vi "Autonomous Independent.vi"   [LabVIEW 2013]
doc: "This VI is called when autonomous begins, and will automatically be terminated when autonomous ends. You can carry out timed or sensor driven robot movement independently without needing to return to the caller."
uses:
  <vilib>/Rock Robotics/WPI/Solenoid/WPI_SolenoidValue.ctl
  Robot Global Data.vi
  <vilib>/Rock Robotics/WPI/RobotDrive/WPI_RobotDriveGetSetRefNum.vi
  <vilib>/Rock Robotics/WPI/Solenoid/WPI_SolenoidSetEnum.vi
  <vilib>/Rock Robotics/WPI/RobotDrive/WPI_RobotDriveArcadeDrive_Standard(NoSaturation).vi
  <vilib>/Rock Robotics/WPI/Solenoid/Deprecated/WPI_SolenoidGetBool.vi
  <vilib>/Rock Robotics/WPI/Joystick/WPI_JoystickGetSetRefNum.vi
panel:
  # "Be sure to right-click and choose Data Operations>>Make Current Value default if you want to save the array values with the VI"
types:
  T1 = typedef "WPI_JoystickDevRef.ctl" = cluster{"Device":T2}
  T2 = typedef "WPI_JoystickDeviceEnum.ctl" = enum16{"USB 1", "USB 2", "USB 3", "USB 4", "Kinect 1", "Kinect 2"}
  T3 = cluster{"axis 1 (x)":dbl, "axis 2 (y)":dbl, "axis 3 (throttle)":dbl, "axis 4":dbl, "axis 5":dbl, "axis 6":dbl}
  T4 = typedef "WPI_MotorControlDeviceRef.ctl" = cluster{"DeviceStatus":errorcluster, "Type":enum16{"PWM", "CAN"}, "PWM":cluster{"Digital Module":T5, "PWM Channel":T6, "DeadBand":T7}, "CAN":cluster{"Device Number":u8, "Control Mode":T8, "Semaphore":T9, "Max Vout":dbl}, "Invert":bool, "TransformRef":T10, "InvTransformRef":T10}
  T5 = typedef "FPGA_TypedefDigitalModule.ctl" = enum16{"Digital Module 1", "Digital Module 2"}
  T6 = typedef "FPGA_DIOPWMChannel.ctl" = enum8{"PWM 1", "PWM 2", "PWM 3", "PWM 4", "PWM 5", "PWM 6", "PWM 7", "PWM 8", "PWM 9", "PWM 10", "Invalid"}
  T7 = typedef "WPI_PWMDeadband.ctl" = cluster{"Name":string, "maxPositivePwm":i32, "minPositivePwm":i32, "centerPwm":i32, "maxNegativePwm":i32, "minNegativePwm":i32, "angularRange":u16}
  T8 = typedef "WPI_CANJaguar_ControlMode.ctl" = enum8{"Percent VBus", "Current", "Speed", "Position", "Voltage"}
  T9 = typedef "Semaphore RefNum" = refnum<k1>
  T10 = typedef "WPI_PWMTransform_ConPane.ctl" = refnum<vi>
  T11 = typedef "WPI_SolenoidDevRef.ctl" = cluster{"DevStatus":errorcluster, "Solenoid Module":T12, "Forward Solenoid Channel":T13, "Reverse Solenoid Channel":T13}
  T12 = typedef "FPGA_TypedefSolenoidModule.ctl" = enum16{"Solenoid Module 1", "Solenoid Module 2"}
  T13 = typedef "WPI_SolenoidChannel.ctl" = enum8{"Solenoid 1", "Solenoid 2", "Solenoid 3", "Solenoid 4", "Solenoid 5", "Solenoid 6", "Solenoid 7", "Solenoid 8", "Invalid"}
  T14 = typedef "WPI_RobotDriveDevRef.ctl" = cluster{"DevStatus":errorcluster, "Motors[]":T4[], "Square Inputs":bool, "Max Output":dbl, "Isochronous":bool}
  T15 = typedef "WPI_SolenoidValue.ctl" = enum16{"Off", "On", "Forward", "Reverse"}
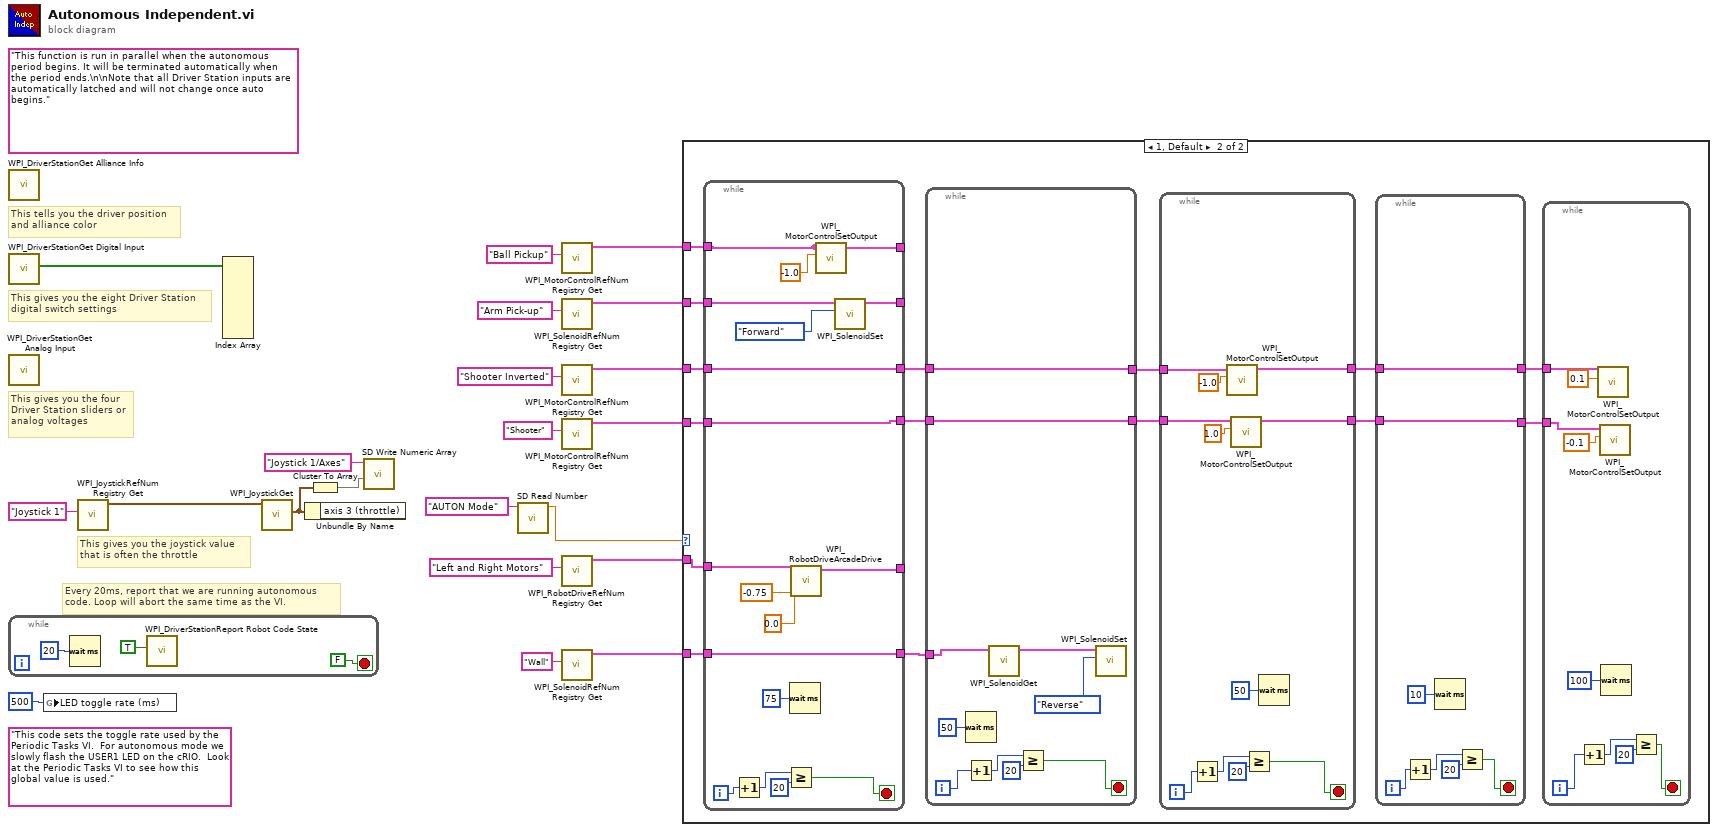
[diagram p0: block diagram]
diagram:
  (unwired) "This code sets the toggle rate used by the Periodic Tasks VI.  For autonomous mode we slowly flash the USER1 LED on the cRIO.  Look at the Periodic Tasks VI to see how this global value is used."
  (unwired) "This function is run in parallel when the autonomous period begins. It will be terminated automatically when the period ends.\n\nNote that all Driver Station inputs are automatically latched and will not change once auto begins."
  # "Every 20ms, report that we are running autonomous\ncode. Loop will abort the same time as the VI."
  # "This gives you the joystick value\nthat is often the throttle"
  # "This tells you the driver position\nand alliance color"
  # "This gives you the eight Driver Station\ndigital switch settings"
  # "This gives you the four\nDriver Station sliders or\nanalog voltages"
  n1 = call <vilib>:"WPI_DriverStationGet Alliance Info.vi"() -> ()  [unwired: 12 out]
  n2 = call <vilib>:"WPI_DriverStationGet Digital Input.vi"() -> ("Driver Station Digital Input (1-8)"=w21:bool[])  [unwired: 11 out]
  n3 = call <vilib>:"WPI_DriverStationGet Analog Input.vi"() -> ()  [unwired: 12 out]
  n4 = while {
    stop <- FALSE stop-if-true
    n5 = Wait (ms)(milliseconds to wait=u32 20) -> ()  [unwired: 1 out]
    n6 = call <vilib>:"WPI_DriverStationReport Robot Code State.vi"("Autonomous"=TRUE) -> ()  [unwired: 10 in, 1 out]
  }
  n7 = global write "Robot Global Data.vi" "LED toggle rate (ms)"(u32 500 ("LED ms toggle rate")) -> ()
  n8 = call <vilib>:"WPI_JoystickRefNum Registry Get.vi"("refnum name"="Joystick 1") -> ("JoystickDevRef"=w19:T1)  [unwired: 1 in, 9 out]
  n9 = Index Array(array=w21) -> ()  [unwired: 8 in, 8 out]
  n10 = call <vilib>:"WPI_JoystickGet.vi"("JoystickDevRef"=w19) -> ("Axes"=w16:T3)  [unwired: 1 in, 5 out]
  n11 = Unbundle By Name(w16) -> ()  [unwired: 1 out]
  n12 = Cluster To Array(cluster=w16) -> (array=w17:dbl[])
  n13 = call <vilib>:"SD Write Numeric Array.vi"("Numeric Array"=w17, "Name"="Joystick 1/Axes") -> ()  [unwired: 8 in, 2 out]
  n14 = call <vilib>:"SD Read Number.vi"("Name"="AUTON Mode") -> ("Numeric"=w13:dbl)  [unwired: 8 in, 2 out]
  n15 = call <vilib>:"WPI_MotorControlRefNum Registry Get.vi"("refnum name"="Ball Pickup") -> ("MotorControlDevRef"=w1:T4)  [unwired: 9 in, 1 out]
  n16 = call <vilib>:"WPI_SolenoidRefNum Registry Get.vi"("refnum name"="Arm Pick-up") -> ("SolenoidDevRef"=w2:T11)  [unwired: 9 in, 1 out]
  n17 = call <vilib>:"WPI_MotorControlRefNum Registry Get.vi"("refnum name"="Shooter Inverted") -> ("MotorControlDevRef"=w3:T4)  [unwired: 9 in, 1 out]
  n18 = call <vilib>:"WPI_MotorControlRefNum Registry Get.vi"("refnum name"="Shooter") -> ("MotorControlDevRef"=w4:T4)  [unwired: 9 in, 1 out]
  n19 = call <vilib>:"WPI_RobotDriveRefNum Registry Get.vi"("refnum name"="Left and Right Motors") -> ("RobotDriveDevRef"=w6:T14)  [unwired: 9 in, 1 out]
  n20 = call <vilib>:"WPI_SolenoidRefNum Registry Get.vi"("refnum name"="Wall") -> ("SolenoidDevRef"=w5:T11)  [unwired: 9 in, 1 out]
  n21 = case shown="1, Default" w13 {
    tunnel: w6 -> [_ w39]
    tunnel: w5 -> [_ w25]
    tunnel: w4 -> [_ w38]
    tunnel: w3 -> [_ w37]
    tunnel: w2 -> [_ w36]
    tunnel: w1 -> [_ w35]
    frame 0 {
    }
    frame 1, Default {
      n22 = while {
        tunnel: w39 -> [w88]
        tunnel: [w86] -> _
        tunnel: [w85] -> w34
        tunnel: w38 -> [w85]
        tunnel: w37 -> [w84]
        tunnel: [w84] -> w33
        tunnel: w36 -> [w79]
        tunnel: w35 -> [w78]
        tunnel: [w78] -> _
        tunnel: [w79] -> _
        tunnel: [w81] -> w26
        tunnel: w25 -> [w81]
        i -> [w92]
        stop <- w89 stop-if-true
        n23 = Increment(x=w92) -> (x+1=w91:i32)
        n24 = Greater Or Equal?(x=w91, y=20) -> (x >= y?=w89:bool)
        n25 = Wait (ms)(milliseconds to wait=u32 75) -> ()  [unwired: 1 out]
        n26 = call-poly <vilib>:"WPI_RobotDriveArcadeDrive.vi"("Y axis value"=-0.75, "X axis value"=0.0, "RobotDriveDevRef"=w88) -> ("RobotDriveDevRef"=w86:T14)  [unwired: 6 in, 2 out]
        n27 = call <vilib>:"WPI_MotorControlSetOutput.vi"("Output"=-1.0, "MotorControlDevRef"=w78) -> ()  [unwired: 7 in, 3 out]
        n28 = call-poly <vilib>:"WPI_SolenoidSet.vi"("Value"=WPI_SolenoidValue."Forward", "SolenoidDevRef"=w79) -> ()  [unwired: 8 in, 2 out]
      }
      n29 = while {
        tunnel: w34 -> [w71]
        tunnel: w33 -> [w72]
        tunnel: [w72] -> w32
        tunnel: [w71] -> w31
        tunnel: w26 -> [w69]
        i -> [w74]
        stop <- w73 stop-if-true
        n30 = Wait (ms)(milliseconds to wait=u32 50) -> ()  [unwired: 1 out]
        n31 = Increment(x=w74) -> (x+1=w75:i32)
        n32 = call-poly <vilib>:"WPI_SolenoidGet.vi"("SolenoidDevRef"=w69) -> ("SolenoidDevRef"=w67:T11)  [unwired: 8 in, 2 out]
        n33 = Greater Or Equal?(x=w75, y=20) -> (x >= y?=w73:bool)
        n34 = call-poly <vilib>:"WPI_SolenoidSet.vi"("Value"=WPI_SolenoidValue."Reverse", "SolenoidDevRef"=w67) -> ()  [unwired: 8 in, 2 out]
      }
      n35 = while {
        tunnel: w32 -> [w62]
        tunnel: w31 -> [w61]
        tunnel: [w58] -> w30
        tunnel: [w57] -> w29
        i -> [w64]
        stop <- w63 stop-if-true
        n36 = Increment(x=w64) -> (x+1=w66:i32)
        n37 = call <vilib>:"WPI_MotorControlSetOutput.vi"("Output"=-1.0, "MotorControlDevRef"=w62) -> ("MotorControlDevRef"=w57:T4)  [unwired: 7 in, 2 out]
        n38 = call <vilib>:"WPI_MotorControlSetOutput.vi"("Output"=1.0, "MotorControlDevRef"=w61) -> ("MotorControlDevRef"=w58:T4)  [unwired: 7 in, 2 out]
        n39 = Greater Or Equal?(x=w66, y=20) -> (x >= y?=w63:bool)
        n40 = Wait (ms)(milliseconds to wait=u32 50) -> ()  [unwired: 1 out]
      }
      n41 = while {
        tunnel: w30 -> [w51]
        tunnel: w29 -> [w50]
        tunnel: [w51] -> w27
        tunnel: [w50] -> w28
        i -> [w52]
        stop <- w53 stop-if-true
        n42 = Increment(x=w52) -> (x+1=w54:i32)
        n43 = Wait (ms)(milliseconds to wait=u32 10) -> ()  [unwired: 1 out]
        n44 = Greater Or Equal?(x=w54, y=20) -> (x >= y?=w53:bool)
      }
      n45 = while {
        tunnel: w28 -> [w47]
        tunnel: w27 -> [w48]
        i -> [w42]
        stop <- w41 stop-if-true
        n46 = Increment(x=w42) -> (x+1=w44:i32)
        n47 = call <vilib>:"WPI_MotorControlSetOutput.vi"("Output"=0.1, "MotorControlDevRef"=w47) -> ()  [unwired: 7 in, 3 out]
        n48 = call <vilib>:"WPI_MotorControlSetOutput.vi"("Output"=-0.1, "MotorControlDevRef"=w48) -> ()  [unwired: 7 in, 3 out]
        n49 = Wait (ms)(milliseconds to wait=u32 100) -> ()  [unwired: 1 out]
        n50 = Greater Or Equal?(x=w44, y=20) -> (x >= y?=w41:bool)
      }
    }
  }
